vi "PV MiniTest Miscellaneous.vi"(8 "error in (no error)":errorcluster, 9 "PV MiniTest Miscellaneous - Cluster":T1={"Parameter"=0, "Parameter\nread only<->describe"=FALSE, "Unit adress"=1, "Load factory settings"=0} {"Load factory settings" min=0 max=468 step=1; "Unit adress" min=1 max=255 step=1; "Parameter" items=[" Error acknowledgement (write only)", " Actual error code (read only)", " Load factory settings (write only)", " Unit adress"]}, 10 "Adress of unit":u16=1 max=999 step=1, 11 "VISA session":refnum<visa-resource-name>) -> (0 "error out":errorcluster, 2 "response (data)":string, 3 "dup VISA session":refnum<visa-resource-name>)   [LabVIEW 2016, in "Pfeiffer Vacuum.lvlib"]
doc: "There are 4 parameters available, only one of which can be enabled at a time. \n\n0 - Error acknowledgement (write only) - Para 009\n1 - Actual error code (read only) (default) - Para 303\n2 - Load factory settings (write only) - Para 656 \n3 - Unit adress - Para797\n\nNote: The two controls right of this one will set the appropriate values for the selected parameter. Any settings for an parameter that is not selected will be ignored. If a value is out of range, it will be changed to either the upper or the lower limit of the range."
uses:
  Pfeiffer Vacuum.lvlib
  PV MiniTest Miscellaneous - Cluster.ctl
panel:
  # "(468 = Load)"
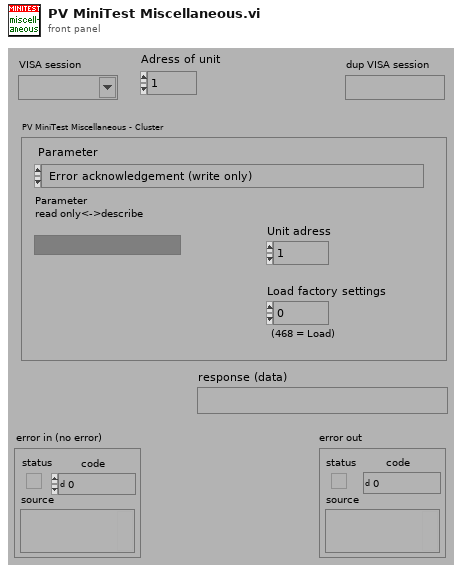
[diagram p1: front panel]
types:
  T1 = typedef "Pfeiffer Vacuum.lvlib/PV MiniTest Miscellaneous - Cluster.ctl" = cluster{"Parameter":u16, "Parameter\nread only<->describe":bool, "Unit adress":i16, "Load factory settings":i16}
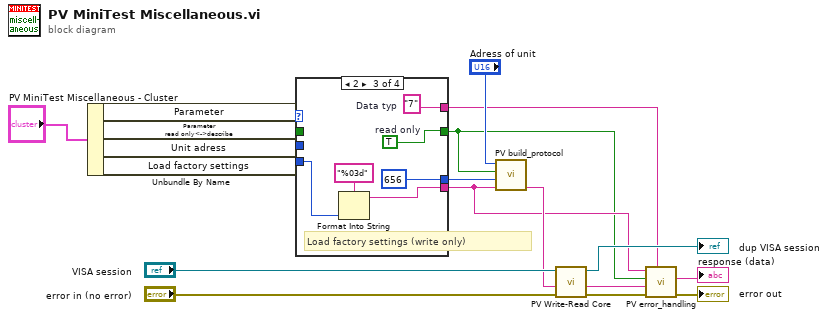
[diagram p0: block diagram]
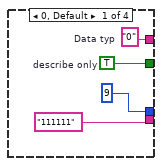
[diagram p2: hidden frame]
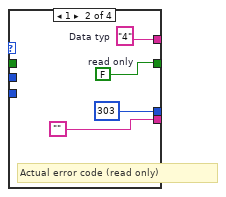
[diagram p3: hidden frame]
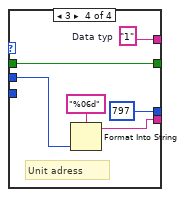
[diagram p4: hidden frame]
diagram:
  n1 = Unbundle By Name("PV MiniTest Miscellaneous - Cluster") -> ("Parameter"=w16:u16, "Parameter\nread only<->describe"=w15:bool, "Unit adress"=w13:i16, "Load factory settings"=w1:i16)
  n2 = case shown="2" w16 {
    tunnel: [u16 9 ("Parameter-number") u16 303 ("Parameter-number") u16 656 ("Parameter-number") u16 797 ("Parameter-number")] -> w17
    tunnel: ["111111" ("Data") "" w28 w37] -> w5
    tunnel: [w22 w25 w31 w35] -> w4
    tunnel: w15 -> [_ _ _ w35]
    tunnel: w13 -> [_ _ _ w34]
    tunnel: [w19 w23 w30 w33] -> w6
    tunnel: w1 -> [_ _ w27 _]
    frame 0, Default {
      w19 = "0"  # Data typ
      w22 = TRUE  # describe only
    }
    frame 1 {
      w23 = "4"  # Data typ
      w25 = FALSE  # read only
      # "Actual error code (read only)"
    }
    frame 2 {
      w30 = "7"  # Data typ
      w31 = TRUE  # read only
      # "Load factory settings (write only)"
      n3 = Format Into String(format string="%03d" ("Format-String"), w27) -> (resulting string=w28:string)  [unwired: 2 in, 1 out]
    }
    frame 3 {
      w33 = "1"  # Data typ
      # "Unit adress"
      n4 = Format Into String(format string="%06d" ("Format-String"), w34) -> (resulting string=w37:string)  [unwired: 2 in, 1 out]
    }
  }
  n5 = call "PV build_protocol.vi"("Data"=w5, "Parameter-number"=w17, "parameter\nread<->describe"=w4, "Adress"="Adress of unit") -> ("output"=w10:string)  [unwired: 3 in]
  n6 = call "PV Write-Read Core.vi"("error in"="error in (no error)", "Write data in"=w10, "VISA session"="VISA session") -> ("error out"=w7:errorcluster, "response (data) out"=w8:string, "dup VISA session"=→"dup VISA session":refnum<visa-resource-name>)  [unwired: 2 in]
  n7 = call "PV error_handling.vi"("Data Typ in"=w6, "error in"=w7, "response (data) in"=w8, "Parameter\nread only<->describe"=w4, "data in"=w5) -> ("error out"=→"error out":errorcluster, "Data out"=→"response (data)":string)  [unwired: 4 in, 1 out]
